vi "Line_Follower_01.vi"() -> ()   [LabVIEW 2014]
uses:
  <vilib>/myRIO/Express VI/Onboard IO/AI/AI Express VI.xnode
  <vilib>/myRIO/Instrument Drivers/Onboard IO/AI/vis/Read.vi
  <vilib>/myRIO/Instrument Drivers/Onboard IO/AI/AI.lvlib
  <vilib>/myRIO/Common/Instrument Driver Framework/Utilities/typedefs/Analog Scaling Constants.ctl
  <vilib>/myRIO/Common/Instrument Driver Framework/Utilities/typedefs/Analog Scaling Constants List.ctl
  <vilib>/myRIO/Common/Instrument Driver Framework/myRIO v1.0/AI/typedefs/AI Channels Enum.ctl
  <vilib>/myRIO/Common/Instrument Driver Framework/myRIO v1.0/AI/typedefs/AI Channels List.ctl
  <vilib>/myRIO/Common/Instrument Driver Framework/Utilities/typedefs/Generic FPGA Reference.ctl
  <vilib>/myRIO/Common/Instrument Driver Framework/Utilities/typedefs/myRIO v1.0 Reference.ctl
  <vilib>/myRIO/Common/Instrument Driver Framework/Utilities/typedefs/Hardware Version Enum.ctl
  <vilib>/myRIO/Common/Instrument Driver Framework/Utilities/typedefs/myRIO Generic Hardware Reference.ctl
  <vilib>/myRIO/Instrument Drivers/Onboard IO/AI/typedefs/AI Reference.ctl
  <vilib>/myRIO/Instrument Drivers/Onboard IO/AI/vis/myRIO AI Open.xnode
  <vilib>/myRIO/Common/Instrument Driver Framework/Utilities/vis/Is FPGA Ref Available.vi
  <vilib>/userdefined/High Color/nirio_resource_hc.ctl
  <vilib>/myRIO/Express VI/Onboard IO/DO/DO Express VI.xnode
  <vilib>/myRIO/Instrument Drivers/Onboard IO/DIO/vis/Write.vi
  <vilib>/myRIO/Instrument Drivers/Onboard IO/DIO/DIO.lvlib
  <vilib>/myRIO/Common/Instrument Driver Framework/myRIO v1.0/DIO/typedefs/DIO Channels Enum.ctl
  <vilib>/myRIO/Common/Instrument Driver Framework/myRIO v1.0/DIO/typedefs/DIO Channels List.ctl
  <vilib>/myRIO/Instrument Drivers/Onboard IO/DIO/typedefs/DIO Reference.ctl
  <vilib>/myRIO/Instrument Drivers/Onboard IO/DIO/vis/myRIO DIO Open.xnode
  <vilib>/myRIO/Common/Instrument Driver Framework/myRIO v1.0/DIO/vis/myRIO v1.1 Open DIO.vi
  <vilib>/myRIO/Common/Instrument Driver Framework/myRIO v1.0/AI/vis/myRIO v1.1 Open AI.vi
panel:
  in  "stop 2":bool
  out "A/AI2 (Pin 7)":dbl
  out "A/AI1 (Pin 5)":dbl
  out "A/AI0 (Pin 3)":dbl
  in  "stop":bool
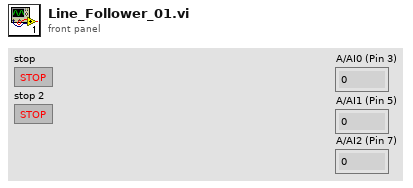
[diagram p1: front panel]
types:
  T1 = typedef "DIO.lvlib/DIO Reference.ctl" = cluster{"myRIO Reference":T2, "DIO Channels List":T6}
  T2 = typedef "myRIO Generic Hardware Reference.ctl" = cluster{"myRIO Model":T3, "myRIO Hardware Reference":T4}
  T3 = typedef "Hardware Version Enum.ctl" = enum16{"Unknown", "myRIO-1900", "myRIO-1950"}
  T4 = typedef "myRIO v1.0 Reference.ctl" = cluster{"Generic FPGA Reference":T5, "Allow multiple opens":bool}
  T5 = typedef "Generic FPGA Reference.ctl" = refnum<k20>
  T6 = typedef "DIO Channels List.ctl" = T7[]
  T7 = typedef "DIO Channels Enum.ctl" = enum16{"Not Connected", "C/DIO0", "C/DIO1", "C/DIO2", "C/DIO3", "C/DIO4", "C/DIO5", "C/DIO6", "C/DIO7", "A/DIO0", "A/DIO1", "A/DIO2", "A/DIO3", "A/DIO4", "A/DIO5", "A/DIO6", "A/DIO7", "A/DIO8", "A/DIO9", "A/DIO10", "A/DIO11", "A/DIO12", "A/DIO13", "A/DIO14", "A/DIO15", "B/DIO0", "B/DIO1", "B/DIO2", "B/DIO3", "B/DIO4", "B/DIO5", "B/DIO6", "B/DIO7", "B/DIO8", "B/DIO9", "B/DIO10", "B/DIO11", "B/DIO12", "B/DIO13", "B/DIO14", "B/DIO15", "LED0", "LED1", "LED2", "LED3", "Button0"}
  T8 = typedef "nirio_resource_hc.ctl" = tag
  T9 = typedef "AI.lvlib/AI Reference.ctl" = cluster{"myRIO Reference":T2, "AI Channels List":T10, "AI Scaling Constants List":T12}
  T10 = typedef "AI Channels List.ctl" = T11[]
  T11 = typedef "AI Channels Enum.ctl" = enum16{"Not Connected", "AudioIn/Left", "AudioIn/Right", "C/AI0", "C/AI1", "A/AI0", "A/AI1", "A/AI2", "A/AI3", "B/AI0", "B/AI1", "B/AI2", "B/AI3"}
  T12 = typedef "Analog Scaling Constants List.ctl" = T13[]
  T13 = typedef "Analog Scaling Constants.ctl" = cluster{"LSB Weight (Volts)":dbl, "Offset (Volts)":dbl, "Signed?":bool}
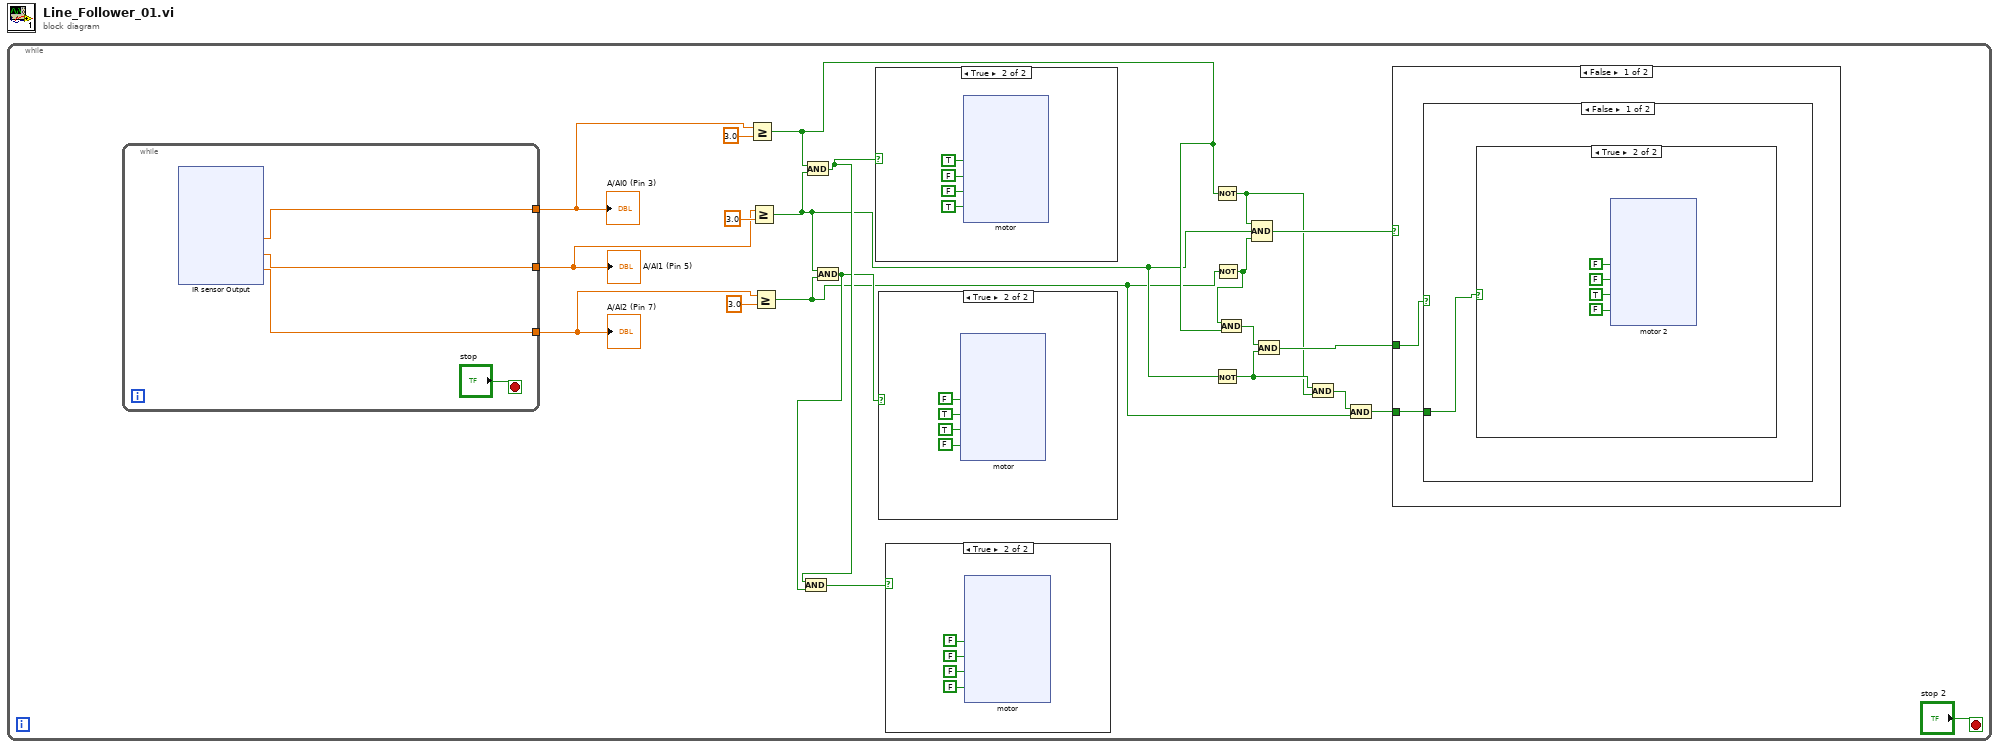
[diagram p0: block diagram]
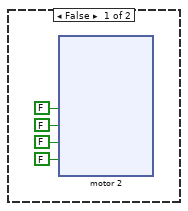
[diagram p2: hidden frame]
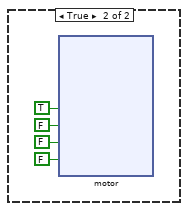
[diagram p3: hidden frame]
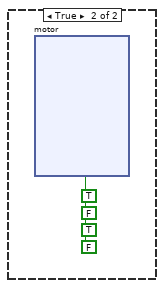
[diagram p4: hidden frame]
diagram:
  n1 = while {
    stop <- "stop 2" stop-if-true
    n2 = while {
      tunnel: [w321] -> w18
      tunnel: [w320] -> w17
      tunnel: [w319] -> w16
      stop <- "stop" stop-if-true
      n3 = xnode "IR sensor Output"() -> ("left (A/AI0 (Pin 3))"=w321:dbl, "middle (A/AI1 (Pin 5))"=w320:dbl, "right (A/AI2 (Pin 7))"=w319:dbl)  [unwired: 1 in, 1 out]
    }
    "A/AI0 (Pin 3)" <- w18
    "A/AI1 (Pin 5)" <- w17
    "A/AI2 (Pin 7)" <- w16
    n4 = Greater Or Equal?(x=w18, y=3.0) -> (x >= y?=w8:bool)
    n5 = Greater Or Equal?(x=w17, y=3.0) -> (x >= y?=w7:bool)
    n6 = Greater Or Equal?(x=w16, y=3.0) -> (x >= y?=w2:bool)
    n7 = And(x=w8, y=w7) -> (x .and. y?=w14:bool)
    n8 = And(x=w7, y=w2) -> (x .and. y?=w13:bool)
    n9 = And(x=w14, y=w13) -> (x .and. y?=w15:bool)
    n10 = case shown="True" w14 {
      frame False {
      }
      frame True {
        n11 = xnode "motor"("m1in1 (A/DIO0 (Pin 11))"=TRUE, "m1in2 (A/DIO1 (Pin 13))"=FALSE, "m2in1 (A/DIO2 (Pin 15))"=FALSE, "m2in2 (A/DIO3 (Pin 17))"=TRUE) -> ()  [unwired: 1 in, 1 out]
      }
    }
    n12 = case shown="True" w13 {
      frame False {
      }
      frame True {
        n13 = xnode "motor "("m1in1 (A/DIO0 (Pin 11))"=FALSE, "m1in2 (A/DIO1 (Pin 13))"=TRUE, "m2in1 (A/DIO2 (Pin 15))"=TRUE, "m2in2 (A/DIO3 (Pin 17))"=FALSE) -> ()  [unwired: 1 in, 1 out]
      }
    }
    n14 = case shown="True" w15 {
      frame False {
      }
      frame True {
        n15 = xnode "motor "("m1in1 (A/DIO0 (Pin 11))"=FALSE, "m1in2 (A/DIO1 (Pin 13))"=FALSE, "m2in1 (A/DIO2 (Pin 15))"=FALSE, "m2in2 (A/DIO3 (Pin 17))"=FALSE) -> ()  [unwired: 1 in, 1 out]
      }
    }
    n16 = Not(x=w8) -> (.not. x?=w3:bool)
    n17 = Not(x=w7) -> (.not. x?=w4:bool)
    n18 = Not(x=w2) -> (.not. x?=w9:bool)
    n19 = And(x=w9, y=w8) -> (x .and. y?=w10:bool)
    n20 = Compound Arithmetic op=AND(w3, w7, w9) -> (w12:bool)
    n21 = And(x=w10, y=w4) -> (x .and. y?=w11:bool)
    n22 = And(x=w4, y=w3) -> (x .and. y?=w6:bool)
    n23 = And(x=w6, y=w2) -> (x .and. y?=w5:bool)
    n24 = case shown="False" w12 {
      tunnel: w11 -> [w23 _]
      tunnel: w5 -> [w22 _]
      frame False {
        n25 = case shown="False" w23 {
          tunnel: w22 -> [w24 _]
          frame False {
            n26 = case shown="True" w24 {
              frame False {
                n27 = xnode "motor 2"("m1in1 (A/DIO0 (Pin 11))"=FALSE, "m1in2 (A/DIO1 (Pin 13))"=FALSE, "m2in1 (A/DIO2 (Pin 15))"=FALSE, "m2in2 (A/DIO3 (Pin 17))"=FALSE) -> ()  [unwired: 1 in, 1 out]
              }
              frame True {
                n28 = xnode "motor 2"("m1in1 (A/DIO0 (Pin 11))"=FALSE, "m1in2 (A/DIO1 (Pin 13))"=FALSE, "m2in1 (A/DIO2 (Pin 15))"=TRUE, "m2in2 (A/DIO3 (Pin 17))"=FALSE) -> ()  [unwired: 1 in, 1 out]
              }
            }
          }
          frame True {
            n29 = xnode "motor "("m1in1 (A/DIO0 (Pin 11))"=TRUE, "m1in2 (A/DIO1 (Pin 13))"=FALSE, "m2in1 (A/DIO2 (Pin 15))"=FALSE, "m2in2 (A/DIO3 (Pin 17))"=FALSE) -> ()  [unwired: 1 in, 1 out]
          }
        }
      }
      frame True {
        n30 = xnode "motor "("m1in1 (A/DIO0 (Pin 11))"=TRUE, "m1in2 (A/DIO1 (Pin 13))"=FALSE, "m2in1 (A/DIO2 (Pin 15))"=TRUE, "m2in2 (A/DIO3 (Pin 17))"=FALSE) -> ()  [unwired: 1 in, 1 out]
      }
    }
  }
